vi "Abort.vi"(8 "error in (no error)":errorcluster, 11 "UI_Interaction_Manager in":refnum<class "UI_Interaction_Manager.lvclass">) -> (0 "error out":errorcluster, 3 "UI_Interaction_Manager out":refnum<class "UI_Interaction_Manager.lvclass">)   [LabVIEW 2011, in "UI_Interaction_Manager.lvclass"]
uses:
  UI_Interaction_Manager.lvclass
  UI_Interaction_Manager.lvclass/UI_Interaction_Manager.ctl
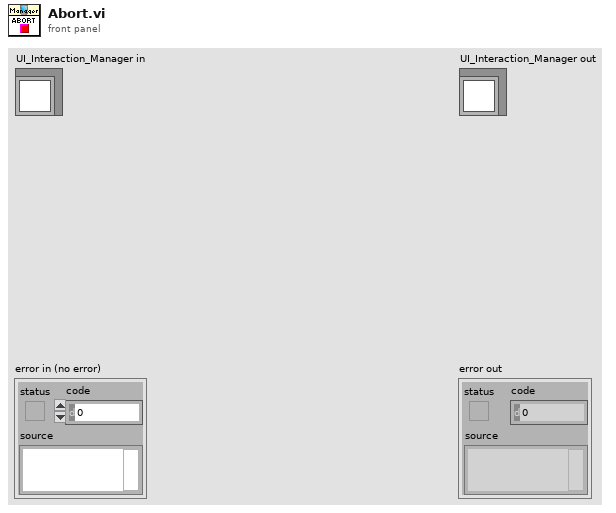
[diagram p1: front panel]
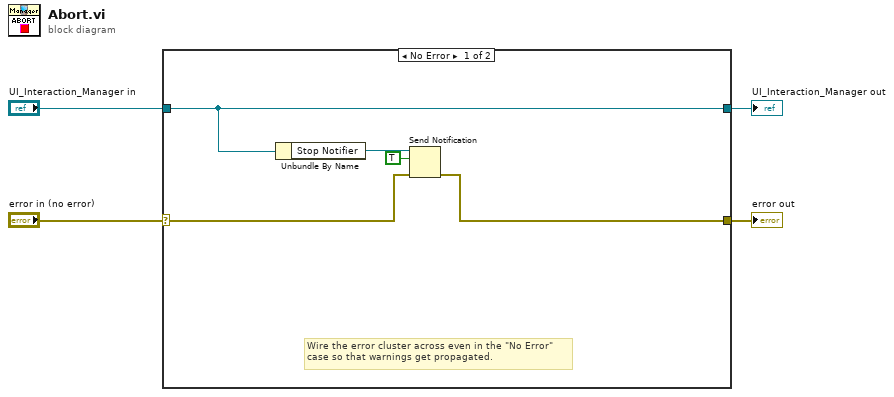
[diagram p0: block diagram]
diagram:
  n1 = case shown="No Error" "error in (no error)" {
    selector: "error in (no error)" -> [w6 w11]
    tunnel: [w5 w11] -> w3
    tunnel: [w8 w10] -> w1
    tunnel: "UI_Interaction_Manager in" -> [w8 w10]
    frame No Error {
      # "Wire the error cluster across even in the \"No Error\"\ncase so that warnings get propagated."
      n2 = Unbundle By Name(w8) -> ("Stop Notifier"=w7:refnum<notifier>)
      n3 = Send Notification(notification=TRUE, notifier=w7, error in (no error)=w6) -> (error out=w5:errorcluster)  [unwired: 1 out]
    }
    frame Error {
    }
  }
  "error out" <- w3
  "UI_Interaction_Manager out" <- w1
